vi "Konwersja_Num_na_Zakr.vi"(10 "Zakres No":i32) -> (2 "Zakres out":enum16{"1000V", "300V", "30V", "3V", "0,3V"}(ring))   [LabVIEW 2014]
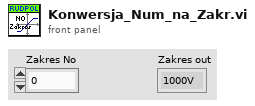
[diagram p1: front panel]
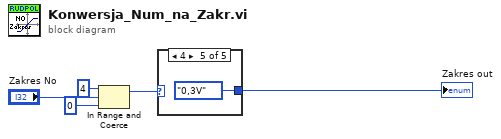
[diagram p0: block diagram]
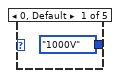
[diagram p2: hidden frame]
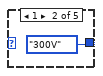
[diagram p3: hidden frame]
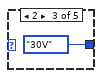
[diagram p4: hidden frame]
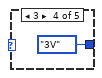
[diagram p5: hidden frame]
diagram:
  n1 = In Range and Coerce(upper limit=4, x="Zakres No", lower limit=0) -> (coerced(x)=w2:i32)  [unwired: 1 out]
  n2 = case shown="4" w2 {
    tunnel: [enum16{"1000V", "300V", "30V", "3V", "0,3V"}."1000V" ("Zakres") enum16{"1000V", "300V", "30V", "3V", "0,3V"}."300V" ("Zakres") enum16{"1000V", "300V", "30V", "3V", "0,3V"}."30V" ("Zakres") enum16{"1000V", "300V", "30V", "3V", "0,3V"}."3V" ("Zakres") enum16{"1000V", "300V", "30V", "3V", "0,3V"}."0,3V" ("Zakres")] -> w1
    frame 0, Default {
    }
    frame 1 {
    }
    frame 2 {
    }
    frame 3 {
    }
    frame 4 {
    }
  }
  "Zakres out" <- w1
